vi "DDC Stage 01 - Single Channel.vi"(10 "ch #":i32, 11 "input cluster":T1={"acq.reset"=FALSE, "data in"=[{"I"=0.0, "Q"=0.0, "overflow"=FALSE}, {"I"=0.0, "Q"=0.0, "overflow"=FALSE}, {"I"=0.0, "Q"=0.0, "overflow"=FALSE}, {"I"=0.0, "Q"=0.0, "overflow"=FALSE}, {"I"=0.0, "Q"=0.0, "overflow"=FALSE}, {"I"=0.0, "Q"=0.0, "overflow"=FALSE}, {"I"=0.0, "Q"=0.0, "overflow"=FALSE}, {"I"=0.0, "Q"=0.0, "overflow"=FALSE}], "input valid"=FALSE, "ddc.freq.shift"=[0.0, 0.0, 0.0, 0.0, 0.0, 0.0, 0.0, 0.0, 0.0, 0.0, 0.0, 0.0, 0.0, 0.0, 0.0, 0.0], "ddc.phase"=[0.0, 0.0, 0.0, 0.0, 0.0, 0.0, 0.0, 0.0, 0.0, 0.0, 0.0, 0.0, 0.0, 0.0, 0.0, 0.0]} {"ddc.freq.shift" format="%.48g"; "ddc.phase" format="%.21g"}) -> (3 "output":T3)   [LabVIEW 2015, in "DDC_7976R_v1.lvlib"]
uses:
  DDC_7976R_v1.lvlib
  Typedef - internal -02.ctl
  Typedef - internal -01.ctl
  <instrlib>/_niInstr/DSP/v1/Shared/Public/IQ Data.ctl
  <instrlib>/_niInstr/DSP/v1/FPGA/Public/Sub VIs/Frequency Shift/Frequency Shift - 8 spc.vi
  <instrlib>/_niInstr/DSP/v1/Xnodes/Public/Frequency Shift/niInstr DSP v1 Frequency Shift FPGA.xnode
  <instrlib>/_niInstr/DSP/v1/Shared/niInstr DSP v1 Shared.lvlib
  <instrlib>/_niInstr/DSP/v1/FPGA/niInstr DSP v1 FPGA.lvlib
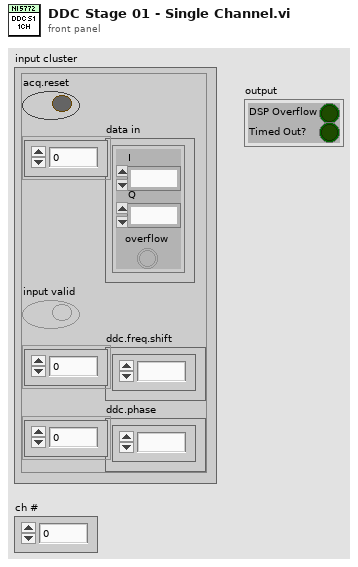
[diagram p1: front panel]
types:
  T1 = typedef "DDC_7976R_v1.lvlib/Typedef - internal -01.ctl" = cluster{"acq.reset":bool, "data in":T2[], "input valid":bool, "ddc.freq.shift":fxp<+/-,48,0>[], "ddc.phase":fxp<+/-,21,0>[]}
  T2 = typedef "niInstr DSP v1 Shared.lvlib/IQ Data.ctl" = cluster{"I":fxp<+/-,18,1>, "Q":fxp<+/-,18,1>, "overflow":bool}
  T3 = typedef "DDC_7976R_v1.lvlib/Typedef - internal -02.ctl" = cluster{"DSP Overflow":bool, "Timed Out?":bool}
  T4 = typedef "DDC_7976R_v1.lvlib/16xIQData.ctl" = T2[]
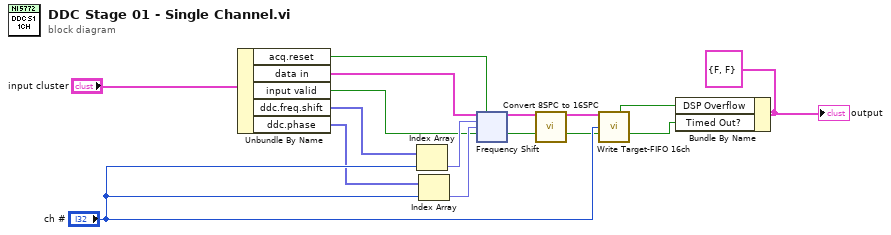
[diagram p0: block diagram]
diagram:
  w16 = T3 {"DSP Overflow"=FALSE, "Timed Out?"=FALSE} ("output cluster")
  n1 = Unbundle By Name("input cluster") -> ("acq.reset"=w7:bool, "data in"=w6:T2[], "input valid"=w5:bool, "ddc.freq.shift"=w4:fxp<+/-,48,0>[], "ddc.phase"=w3:fxp<+/-,21,0>[])
  n2 = Index Array(array=w4, index="ch #") -> (element=w11:fxp<+/-,48,0>)
  n3 = Index Array(array=w3, index="ch #") -> (element=w10:fxp<+/-,21,0>)
  n4 = xnode "Frequency Shift"("data in"=w6, "reset"=w7, "frequency shift"=w11, "phase"=w10, "input valid"=w5) -> ("data out"=w12:T2[], "output valid"=w13:bool)  [unwired: 1 in, 1 out]
  n5 = call "Convert 8SPC to 16SPC.vi"("8xIQ in"=w12, "input valid"=w13) -> ("16xIQ out"=w8:T4, "output valid"=w9:bool)  [unwired: 12 in]
  n6 = call "Write Target-FIFO 16ch.vi"("16xIQ in"=w8, "Ch select"="ch #", "input valid"=w9) -> ("DSP Overflow"=w2:bool, "Timed Out?"=w1:bool)  [unwired: 11 in]
  n7 = Bundle By Name(cluster=w16, "DSP Overflow"=w2, "Timed Out?"=w1) -> ()  [unwired: 1 out]
  "output" <- w16
